vi "I2C GestureSensor PAJ7620U2.vi"() -> ()   [LabVIEW 2020, in "CTI-Scratchpad.lvlib"]
uses:
  CTI-Scratchpad.lvlib
  CTI/Identity.ctl
  CTI/Error Reporting.ctl
  CTI/GPIO Number.ctl
  CTI/I2C Number.ctl
  CTI/Session/Session.lvclass
  CTI-Peripheral/Gesture Sensor/Grove Gesture Sensor PAJ7620U2/Grove Gesture Sensor PAJ7620U2.lvclass
  CTI/VisaComms/VisaComms.lvclass
  CTI/CTI.lvlib
panel:
  out "Pict Ring":u16(ring)
  out "loop":i32
  in  "stop":bool
  out "Identity":T1
  in  "Grove Connector":enum16{"I2C0", "I2C1"}(ring)
  out "error out":errorcluster
  in  "Port":refnum<visa-resource-name>="COM4"
  # "https://www.seeedstudio.com/Grove-Gesture-PAJ7620U2.html"
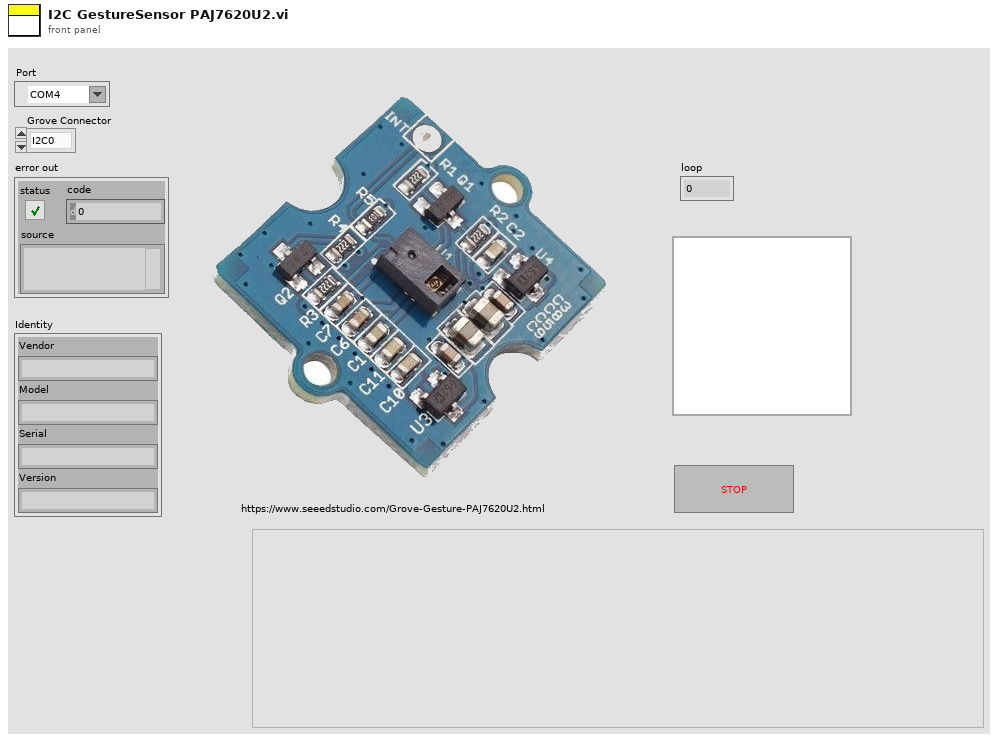
[diagram p1: front panel]
types:
  T1 = typedef "CTI.lvlib/Identity.ctl" = cluster{"Vendor":string, "Model":string, "Serial":string, "Version":string}
  T2 = typedef "CTI.lvlib/Error Reporting.ctl" = enum16{"Minimal", "Moderate", "Full"}
  T3 = typedef "CTI.lvlib/I2C Number.ctl" = i8
  T4 = typedef "CTI.lvlib/GPIO Number.ctl" = i8
  T5 = typedef "CTI-Peripheral.lvlib/Gesture Sensor.lvclass/Gesture.ctl" = enum16{"No Gesture", "Up", "Down", "Left", "Right", "Forward", "Backward", "Clockwise", "Counterclockwise", "Wave"}
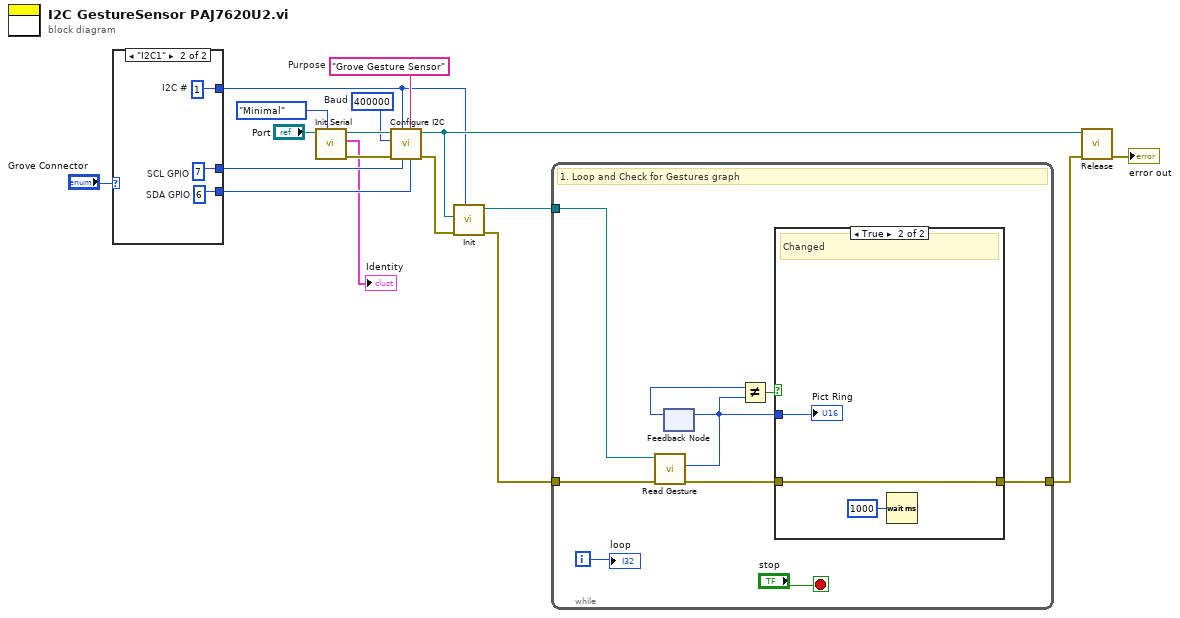
[diagram p0: block diagram]
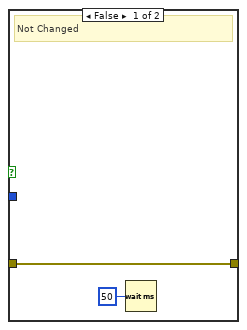
[diagram p2: hidden frame]
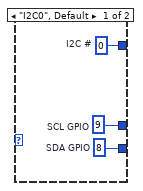
[diagram p3: hidden frame]
diagram:
  w12 = "Grove Gesture Sensor"  # Purpose
  w13 = u32 400000  # Baud
  n1 = case shown="\"I2C1\"" "Grove Connector" {
    tunnel: [w20 w23] -> w8
    tunnel: [w19 w22] -> w7
    tunnel: [w18 w21] -> w6
    frame "I2C0", Default {
      w18 = T3 0  # I2C #
      w19 = T4 8  # SDA GPIO
      w20 = T4 9  # SCL GPIO
    }
    frame "I2C1" {
      w21 = T3 1  # I2C #
      w22 = T4 6  # SDA GPIO
      w23 = T4 7  # SCL GPIO
    }
  }
  n2 = call "Init Serial.vi"("Error Checking (Full)"=Error_Reporting."Minimal", "VISA resource name in"="Port") -> ("error out"=w14:errorcluster, "Identity"=→"Identity":T1, "Session"=w15:refnum<class "Session.lvclass">)  [unwired: 7 in]
  n3 = call "Configure I2C.vi"("SDA GPIO"=w7, "Purpose (\"I2C\")"=w12, "SCL GPIO"=w8, "I2C #"=w6, "error in (no error)"=w14, "Baud"=w13, "Session in"=w15) -> ("error out"=w11:errorcluster, "Session out"=w10:refnum<class "Session.lvclass">)  [unwired: 3 in]
  n4 = call "Init.vi"("I2C #"=w6, "error in (no error)"=w11, "Session In"=w10) -> ("error out"=w3:errorcluster, "Grove Gesture Sensor PAJ7620U2 Out"=w4:refnum<class "Grove Gesture Sensor PAJ7620U2.lvclass">)  [unwired: 7 in]
  n5 = while {
    tunnel: w3 -> [w30]
    tunnel: w4 -> [w31]
    tunnel: [w26] -> w2
    i -> [w29]
    stop <- "stop" stop-if-true
    # "1. Loop and Check for Gestures graph"
    n6 = call-dynamic "Read Gesture.vi"("error in (no error)"=w30, "Grove Gesture Sensor PAJ7620U2 in"=w31) -> ("error out"=w27:errorcluster, "Gesture"=w24:T5)  [unwired: 7 in, 1 out]
    n7 = feedback-in #1(w24) -> ()
    n8 = feedback #1() -> (w28:T5)  [unwired: 1 in]
    n9 = Not Equal?(x=w28, y=w24) -> (x != y?=w25:bool)
    n10 = case shown="True" w25 {
      tunnel: w27 -> [w33 w36]
      tunnel: [w33 w36] -> w26
      tunnel: w24 -> [_ w35]
      frame False {
        # "Not Changed"
        n11 = Wait (ms)(milliseconds to wait=u32 50) -> ()  [unwired: 1 out]
      }
      frame True {
        # "Changed"
        n12 = Wait (ms)(milliseconds to wait=u32 1000) -> ()  [unwired: 1 out]
        "Pict Ring" <- w35
      }
    }
    "loop" <- w29
  }
  n13 = call-dynamic "Release.vi"("error in (no error)"=w2, "Session in"=w10) -> ("error out"=→"error out":errorcluster)  [unwired: 9 in]
